vi "Set FPGA Bitfile Path.vi"(10 "FPGA Bitfile Path":path, 11 "Scalar Channels Testing in":refnum<class "FPGA Addon Test Class.lvclass">) -> (3 "Scalar Channels Testing out":refnum<class "FPGA Addon Test Class.lvclass">)   [LabVIEW 2019, in "FPGA Addon Test Class.lvclass"]
uses:
  FPGA Addon Test Class.lvclass
  FPGA Addon Test Class.lvclass/FPGA Addon Test Class.ctl
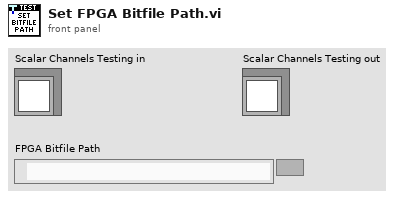
[diagram p1: front panel]
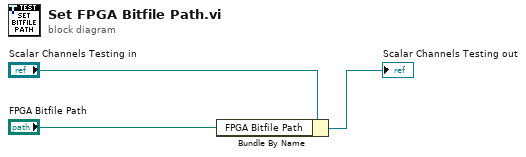
[diagram p0: block diagram]
diagram:
  n1 = Bundle By Name(cluster="Scalar Channels Testing in", "FPGA Bitfile Path"="FPGA Bitfile Path") -> (→"Scalar Channels Testing out":refnum<class "FPGA Addon Test Class.lvclass">)
